vi "Actor Core.vi"(8 "error in":errorcluster, 11 "Nested in":refnum<class "Dinero.lvclass">) -> (0 "error out":errorcluster, 3 "Actor out":refnum<class "Actor.lvclass">)   [LabVIEW 2020, in "Dinero.lvlib" / "Dinero.lvclass"]
doc: "(<B>Filename</B>: Actor Framework.lvlib:Actor.lvclass:Actor Core.vi)\n\nReceives messages to the actor, reacts to them, and initiates any error handling that may shut the actor down.\n\nDescendant classes may override this VI to append parallel tasks for the actor to complete while it handles messages. Overrides use the Call Parent Method node."
uses:
  Dinero.lvclass
  C:/Program Files (x86)/National Instruments/LabVIEW 2020/vi.lib/ActorFramework/Actor/Actor.lvclass
  <vilib>/ActorFramework/Actor/Actor.lvclass
  <vilib>/ActorFramework/Actor/Actor.lvclass/Actor.ctl
  <vilib>/ActorFramework/Message Enqueuer/Message Enqueuer.lvclass/Message Enqueuer.ctl
  Dinero.lvclass/Dinero.ctl
  Dinero Messages/Credit Msg/Credit Msg.lvclass/Credit Msg.ctl
  <vilib>/ActorFramework/Message Enqueuer/Init from Existing Queue.vi
  <vilib>/ActorFramework/Message Enqueuer/Enqueue.vi
  <vilib>/ActorFramework/Stop Msg/Stop Msg.lvclass
  C:/Program Files (x86)/National Instruments/LabVIEW 2020/vi.lib/ActorFramework/Message/Message.lvclass
  Dinero Messages/Credit Msg/Credit Msg.lvclass
  <vilib>/ActorFramework/Message Priority Queue/Priority Enqueue.vi
  <vilib>/ActorFramework/Message Enqueuer/Message Enqueuer.lvclass
panel:
  in  "Monedas":T1
  in  "Change":dbl format="$%.1f"
  in  "Credit":dbl format="$%.1f"
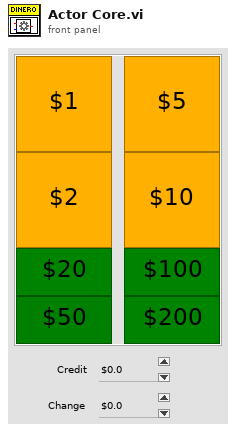
[diagram p1: front panel]
types:
  T1 = cluster{"Moneda 1":bool, "Moneda 2":bool, "Moneda 5":bool, "Moneda 10":bool, "Billete 20":bool, "Billete 50":bool, "Billete 100":bool, "Billete 200":bool}
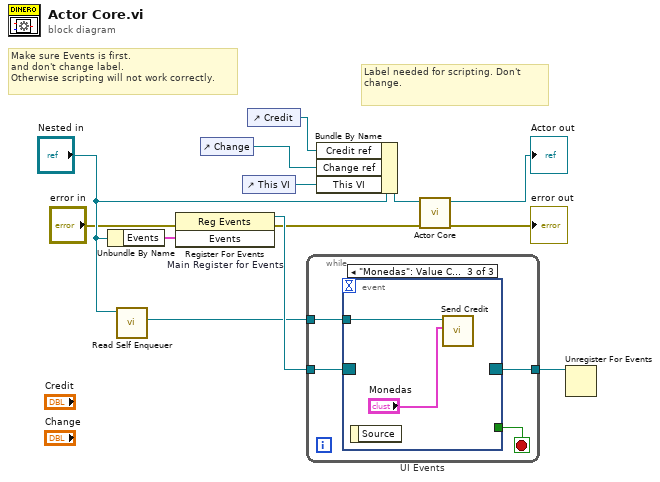
[diagram p0: block diagram]
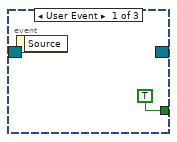
[diagram p2: hidden frame]
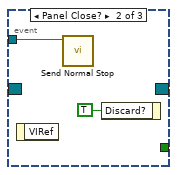
[diagram p3: hidden frame]
diagram:
  # "Label needed for scripting. Don't change."
  # "Make sure Events is first.\nand don't change label.\nOtherwise scripting will not work correctly."
  n1 = Unbundle By Name("Nested in") -> ("Events"=w10:cluster{"Stop":refnum<user-event>})
  n2 = call <vilib>:"Read Self Enqueuer.vi"("Actor"="Nested in") -> ("Self Enqueuer"=w7:refnum<class "Message Enqueuer.lvclass">)  [unwired: 10 in]
  n3 = register-events "Main Register for Events"(error in="error in", w10) -> (reference out=w11:refnum<event-registration>, error out=w5:errorcluster)  [unwired: 1 in]
  n4 = control-ref of="Change"() -> (w1:refnum<vi>)
  n5 = control-ref of="This VI"() -> (w3:refnum<vi>)
  n6 = control-ref of="Credit"() -> (w2:refnum<vi>)
  n7 = while {
    tunnel: w11 -> [w17]
    tunnel: [w15] -> w9
    tunnel: w7 -> [w14]
    stop <- w16 stop-if-true
    n8 = event "UI Events" shown="[2] \"Monedas\": Value Change" {
      selector: w17 -> [_ _ _]
      dyn-events: [_ _ _] -> w15
      timeout: _ -> [_ _ _]
      tunnel: [TRUE _ _] -> w16
      tunnel: w14 -> [_ w19 w22]
      event User Event {
        n9 = event-data() -> ()  [unwired: 1 in, 1 out]
      }
      event Panel Close? {
        n10 = event-data() -> ()  [unwired: 1 in, 1 out]
        n11 = call <vilib>:"Send Normal Stop.vi"("Message Enqueuer"=w19) -> ()  [unwired: 10 in, 1 out]
        n12 = event-data("Discard?"=TRUE) -> ()  [unwired: 1 in, 1 out]
      }
      event "Monedas": Value Change {
        n13 = event-data() -> ()  [unwired: 1 in, 1 out]
        n14 = call "Send Credit.vi"("Monedas"="Monedas", "Message Enqueuer"=w22) -> ()  [unwired: 8 in, 2 out]
      }
    }
  }
  n15 = Bundle By Name(cluster="Nested in", "Credit ref"=w2, "Change ref"=w1, "This VI"=w3) -> (w4:refnum<class "Dinero.lvclass">)
  n16 = call-parent "Actor Core.vi"("error in"=w5, "Actor in"=w4) -> ("error out"=→"error out":errorcluster, "Actor out"=→"Actor out":refnum<class "Actor.lvclass">)  [unwired: 8 in]
  n17 = Unregister For Events(event registration refnum=w9) -> ()  [unwired: 1 in, 1 out]
